vi "SParam RFSG De-embedding.vi"(8 "error in":errorcluster, 10 "RFmxVNA Settings":T2={"VST Resource Name"="VNA-5633", "RFSG Port"="", "RFmx Port"="", "RF Out Switch"="VNA-5633", "RF Out Connection"={"Common RFout"="", "Port1 Incident"="", "Port2 Incident"=""}, "RF In Switch"="VNA-5633", "RF In Connection"={"Common RFin"="", "Port1 Reference"="", "Port1 Test"="", "Port2 Reference"="", "Port2 Test"=""}, "RFSG attenuation mode"=enum."Constant Attenuation", "RFSG Constant Attenuation (dB)"=0.0, "Save Calibration File at"=path "", "Short S1P"=path "", "Open S1P"=path "", "Load S1P"=path "", "Through Adapter S2P"=path ""}, 11 "S-Par Reference In":T1) -> (0 "error out":errorcluster, 3 "S-Par Reference Out":T1)   [LabVIEW 2023]
uses:
  Controls/Hardware Config - SParam_VST.ctl
  <vilib>/niSPML/Typedefs/Session Handle.ctl
  <vilib>/niSPML/S-Par Reference.lvclass
  <vilib>/niSPML/Typedefs/RFSG Attenuation Path Selection.ctl
  <vilib>/niSPML/Configure RFSG Attenuation (Constant).vi
  <vilib>/niSPML/S-Parameter Measurements.lvlib
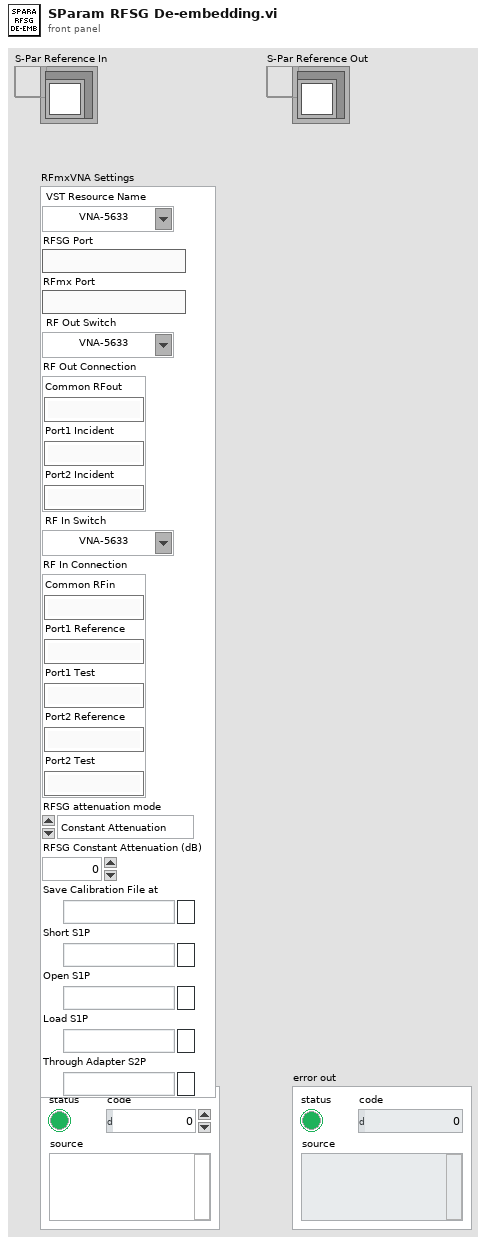
[diagram p1: front panel]
types:
  T1 = typedef "S-Parameter Measurements.lvlib/S-Par Reference.lvclass/Session Handle.ctl" = refnum<data-value>
  T2 = typedef "Hardware Config - SParam_VST.ctl" = cluster{"VST Resource Name":refnum<k15>, "RFSG Port":string, "RFmx Port":string, "RF Out Switch":refnum<k15>, "RF Out Connection":cluster{"Common RFout":string, "Port1 Incident":string, "Port2 Incident":string}, "RF In Switch":refnum<k15>, "RF In Connection":cluster{"Common RFin":string, "Port1 Reference":string, "Port1 Test":string, "Port2 Reference":string, "Port2 Test":string}, "RFSG attenuation mode":enum32{"<None>", "Constant Attenuation"}, "RFSG Constant Attenuation (dB)":dbl, "Save Calibration File at":path, "Short S1P":path, "Open S1P":path, "Load S1P":path, "Through Adapter S2P":path}
  T3 = typedef "S-Parameter Measurements.lvlib/S-Par Reference.lvclass/RFSG Attenuation Path Selection.ctl" = enum16{"Port 1 & Port 2"}
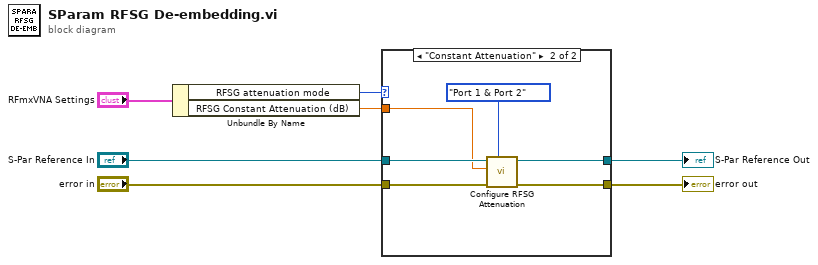
[diagram p0: block diagram]
diagram:
  n1 = Unbundle By Name("RFmxVNA Settings") -> ("RFSG attenuation mode"=w4:enum32{"<None>", "Constant Attenuation"}, "RFSG Constant Attenuation (dB)"=w3:dbl)
  n2 = case shown="\"Constant Attenuation\"" w4 {
    tunnel: "error in" -> [w8 w15]
    tunnel: "S-Par Reference In" -> [w9 w14]
    tunnel: w3 -> [_ w13]
    tunnel: [w9 w12] -> w1
    tunnel: [w8 w11] -> w2
    frame Default {
    }
    frame "Constant Attenuation" {
      n3 = call-poly <vilib>:"Configure RFSG Attenuation.vi"("Path Selection"=RFSG_Attenuation_Path_Selection."Port 1 & Port 2", "error in"=w15, "Tx Constant Attenuation (dB)"=w13, "S-Par Reference In"=w14) -> ("error out"=w11:errorcluster, "S-Par Reference Out"=w12:T1)  [unwired: 6 in]
    }
  }
  "error out" <- w2
  "S-Par Reference Out" <- w1
